vi "AlazarGetWhoTriggeredBySystemHandle.vi"(4 "error in (no error)":errorcluster, 5 "Record Number":u32, 6 "Board ID":u32, 7 "Handle":u64) -> (0 "error out":errorcluster, 2 "Who":u32, 3 "Handle":u64)   [LabVIEW 2018]
doc: "Return which event caused a board system to trigger and capture a record to on-board memory."
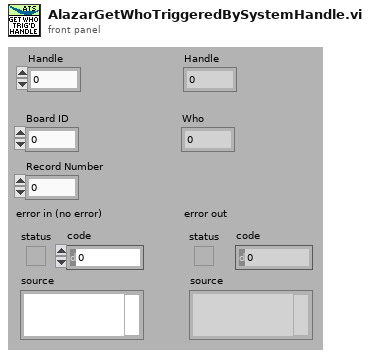
[diagram p1: front panel]
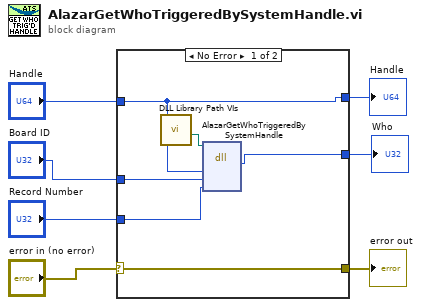
[diagram p0: block diagram]
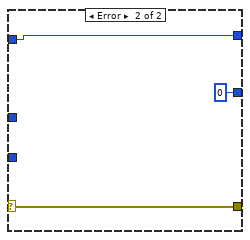
[diagram p2: hidden frame]
diagram:
  n1 = case shown="No Error" "error in (no error)" {
    selector: "error in (no error)" -> [w9 w16]
    tunnel: [w9 w16] -> w6
    tunnel: "Handle" -> [w13 w15]
    tunnel: [w13 w15] -> w4
    tunnel: "Board ID" -> [w12 _]
    tunnel: "Record Number" -> [w11 _]
    tunnel: [w10 0] -> w1
    frame No Error {
      n2 = call "DLL Library Path VIs.vi"() -> ("Alazar"=w8:path)  [unwired: 9 in, 2 out]
      n3 = dll-call lib="C:/Project/SerialSectOCT - FFT GPU/SerialSectOCT/Labview Software/DLL/ATSApi.dll" fn="AlazarGetWhoTriggeredBySystemHandle"(path in=w8, "handle"=w13, "boardID"=w12, "recordNumber"=w11) -> ("return type"=w10:u32)  [unwired: 5 in, 2 out]
    }
    frame Error {
    }
  }
  "Handle" <- w4
  "error out" <- w6
  "Who" <- w1
